vi "Check_Database.vi"(11 "Zip Code":string) -> (2 "Longitude":string, 3 "Temp":string)   [LabVIEW 2014]
uses:
  <vilib>/httpClient/LabVIEWHTTPClient.lvlib
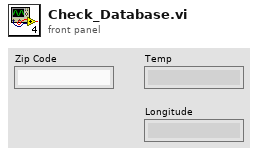
[diagram p1: front panel]
types:
  T1 = typedef "LabVIEWHTTPClient.lvlib/ClientHandle.ctl" = refnum<k1>
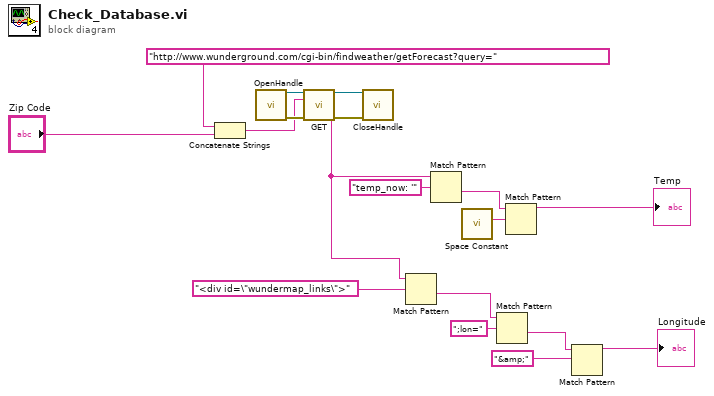
[diagram p0: block diagram]
diagram:
  n1 = Concatenate Strings("http://www.wunderground.com/cgi-bin/findweather/getForecast?query=" ("string"), "Zip Code") -> (w3:string)
  n2 = call <vilib>:"OpenHandle.vi"() -> ("client handle out"=w10:T1, "error out"=w9:errorcluster)  [unwired: 14 in]
  n3 = call <vilib>:"GET.vi"("client handle"=w10, "url"=w3, "error in (no error)"=w9) -> ("client handle out"=w7:T1, "body"=w17:string, "error out"=w8:errorcluster)  [unwired: 9 in, 1 out]
  n4 = call <vilib>:"CloseHandle.vi"("client handle"=w7, "error in (no error)"=w8) -> ()  [unwired: 13 in, 1 out]
  n5 = Match Pattern(string=w17, regular expression="<div id=\"wundermap_links\">") -> (after substring=w18:string)  [unwired: 1 in, 3 out]
  n6 = Match Pattern(string=w17, regular expression="temp_now: '") -> (after substring=w5:string)  [unwired: 1 in, 3 out]
  n7 = call <vilib>:"Space Constant.vi"() -> ("String"=w6:string)
  n8 = Match Pattern(string=w18, regular expression=";lon=") -> (after substring=w13:string)  [unwired: 1 in, 3 out]
  n9 = Match Pattern(string=w5, regular expression=w6) -> (before substring=→"Temp":string)  [unwired: 1 in, 3 out]
  n10 = Match Pattern(string=w13, regular expression="&amp;") -> (before substring=→"Longitude":string)  [unwired: 1 in, 3 out]
